vi "Global_vars.vi"() -> ()   [LabVIEW 2014]
panel:
  in  "Line 2":T1 {"Point2 (Real-World)"."Y" format="%.2f"; "Point2 (Real-World)"."X" format="%.2f"; "Point1 (Real-World)"."Y" format="%.2f"; "Point1 (Real-World)"."X" format="%.2f"; "Point2 (Pixels)"."Y" format="%.2f"; "Point2 (Pixels)"."X" format="%.2f"; "Point1 (Pixels)"."Y" format="%.2f"; "Point1 (Pixels)"."X" format="%.2f"}
  in  "Line 1":T1 {"Point2 (Real-World)"."Y" format="%.2f"; "Point2 (Real-World)"."X" format="%.2f"; "Point1 (Real-World)"."Y" format="%.2f"; "Point1 (Real-World)"."X" format="%.2f"; "Point2 (Pixels)"."Y" format="%.2f"; "Point2 (Pixels)"."X" format="%.2f"; "Point1 (Pixels)"."Y" format="%.2f"; "Point1 (Pixels)"."X" format="%.2f"}
  in  "Vision Map":dbl[][](array[numeric])
  in  "LR Command":dbl
  in  "FR Command":dbl
  in  "STOP":bool
  in  "CompassOut":dbl
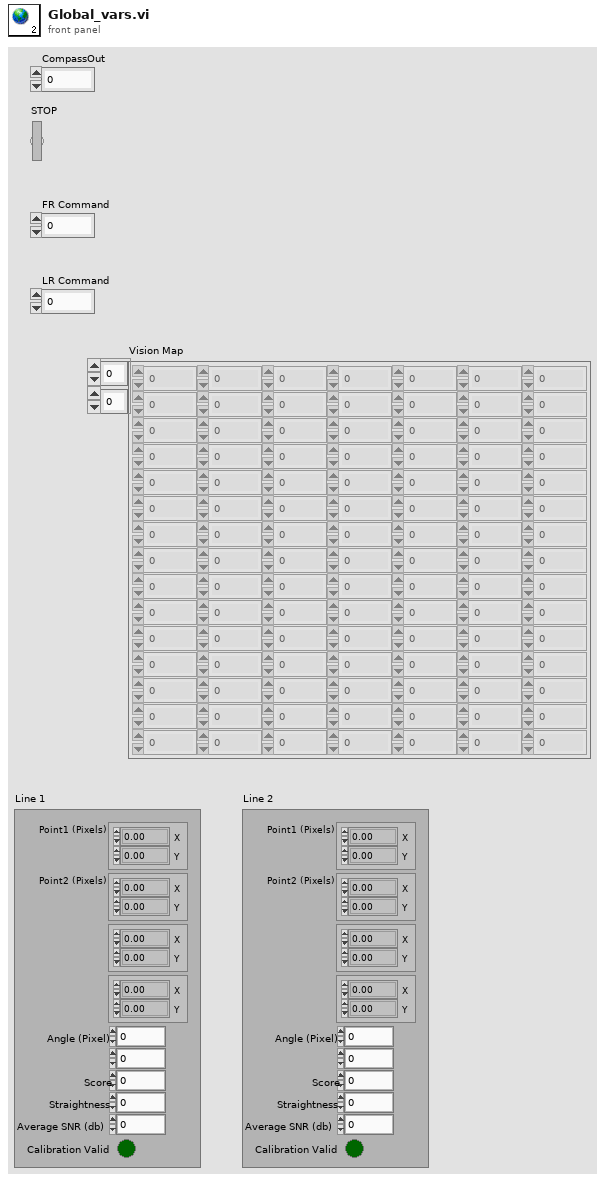
[diagram p1: front panel]
types:
  T1 = cluster{"Point1 (Pixels)":cluster{"X":sgl, "Y":sgl}, "Point2 (Pixels)":cluster{"X":sgl, "Y":sgl}, "Point1 (Real-World)":cluster{"X":sgl, "Y":sgl}, "Point2 (Real-World)":cluster{"X":sgl, "Y":sgl}, "Angle (Pixel)":dbl, "Angle (Real-World)":dbl, "Score":dbl, "Straightness":dbl, "Average SNR (db)":dbl, "Calibration Valid":bool}
diagram:
